vi "Disconnect.vi"(8 "error in (no error)":errorcluster, 11 "H-Intfc in":refnum<class "EnVision REST.lvclass">) -> (0 "error out":errorcluster, 3 "H-Intfc out":refnum<class "EnVision REST.lvclass">)   [LabVIEW 2018, in "EnVision REST.lvlib" / "EnVision REST.lvclass"]
uses:
  EnVision REST.lvclass
  EnVision REST.lvclass/EnVision REST.ctl
  <vilib>/addons/_JKI.lib/REST Client/classes/REST Client/REST Client.lvclass
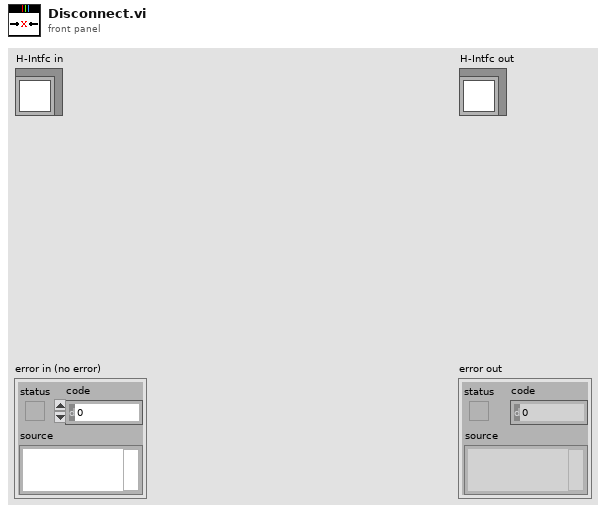
[diagram p1: front panel]
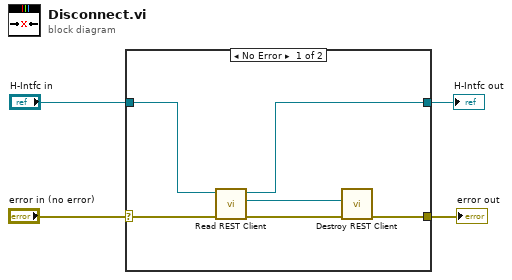
[diagram p0: block diagram]
diagram:
  n1 = case shown="No Error" "error in (no error)" {
    selector: "error in (no error)" -> [w9 w12]
    tunnel: [w6 w12] -> w3
    tunnel: [w5 w11] -> w2
    tunnel: "H-Intfc in" -> [w10 w11]
    frame No Error {
      n2 = call "Read REST Client.vi"("error in (no error)"=w9, "EnVision REST in"=w10) -> ("error out"=w7:errorcluster, "REST Client.lvlib:REST Client.lvclass"=w8:refnum<class "REST Client.lvclass">, "EnVision REST out"=w5:refnum<class "EnVision REST.lvclass">)  [unwired: 7 in]
      n3 = call-dynamic "Destroy REST Client.vi"("error in (no error)"=w7, "REST Client in"=w8) -> ("error out"=w6:errorcluster)  [unwired: 9 in]
    }
    frame Error {
    }
  }
  "error out" <- w3
  "H-Intfc out" <- w2
